vi "AddConstantPotential.vi"(0 "deviceName":string, 1 "channel":u8, 2 "repeats":u16=1, 3 "potential":sgl, 4 "samplingInterval":sgl, 5 "maxDuration":sgl, 6 "isVoltageVsOCP":bool, 7 "error in (no error)":errorcluster, 8 "maxAbsoluteCurrent":sgl=inf, 10 "minAbsoluteCurrent":sgl, 12 "maxCapacity":sgl=inf, 13 "mindIdt":sgl, 14 "approxMaxCurrent":sgl=inf, 15 "isAutoRange":bool=TRUE, 16 "voltageRange":i32=-1) -> (27 "error out":errorcluster)   [LabVIEW 2018]
doc: "EXPORT void AisAddConstantPotential(const char* deviceName, uint8_t channel, uint16_t repeats, float potential, float samplingInterval, float maxDuration, bool isVoltageVsOCP, float maxAbsoluteCurrent, float maxCurrent, float minAbsoluteCurrent, float minCurrent, float maxCapacity, float mindIdt, float approxMaxCurrent, bool isAutoRange, int voltageRange);"
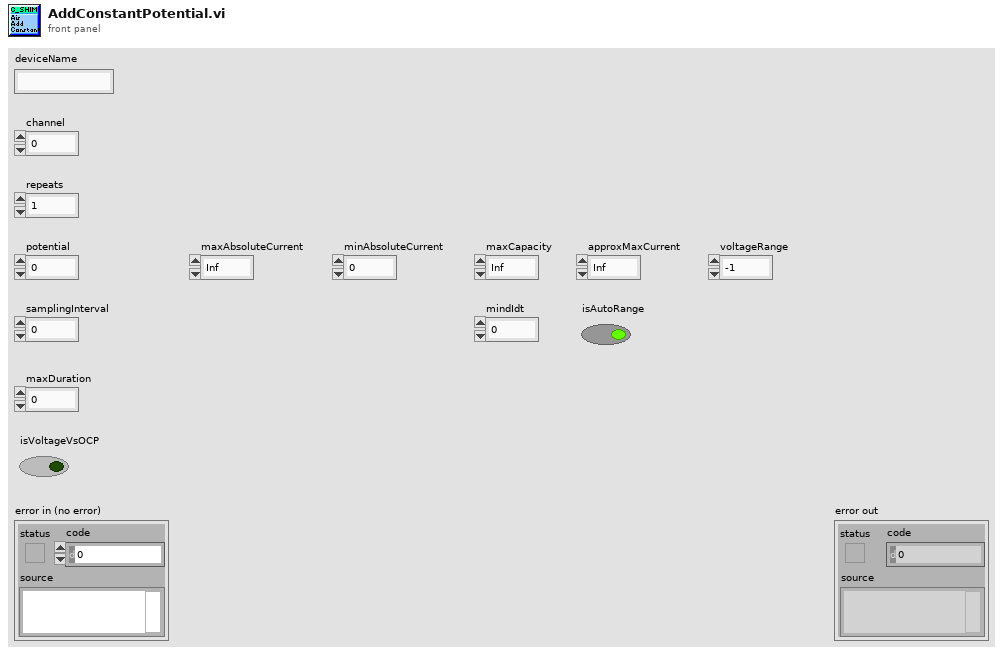
[diagram p1: front panel]
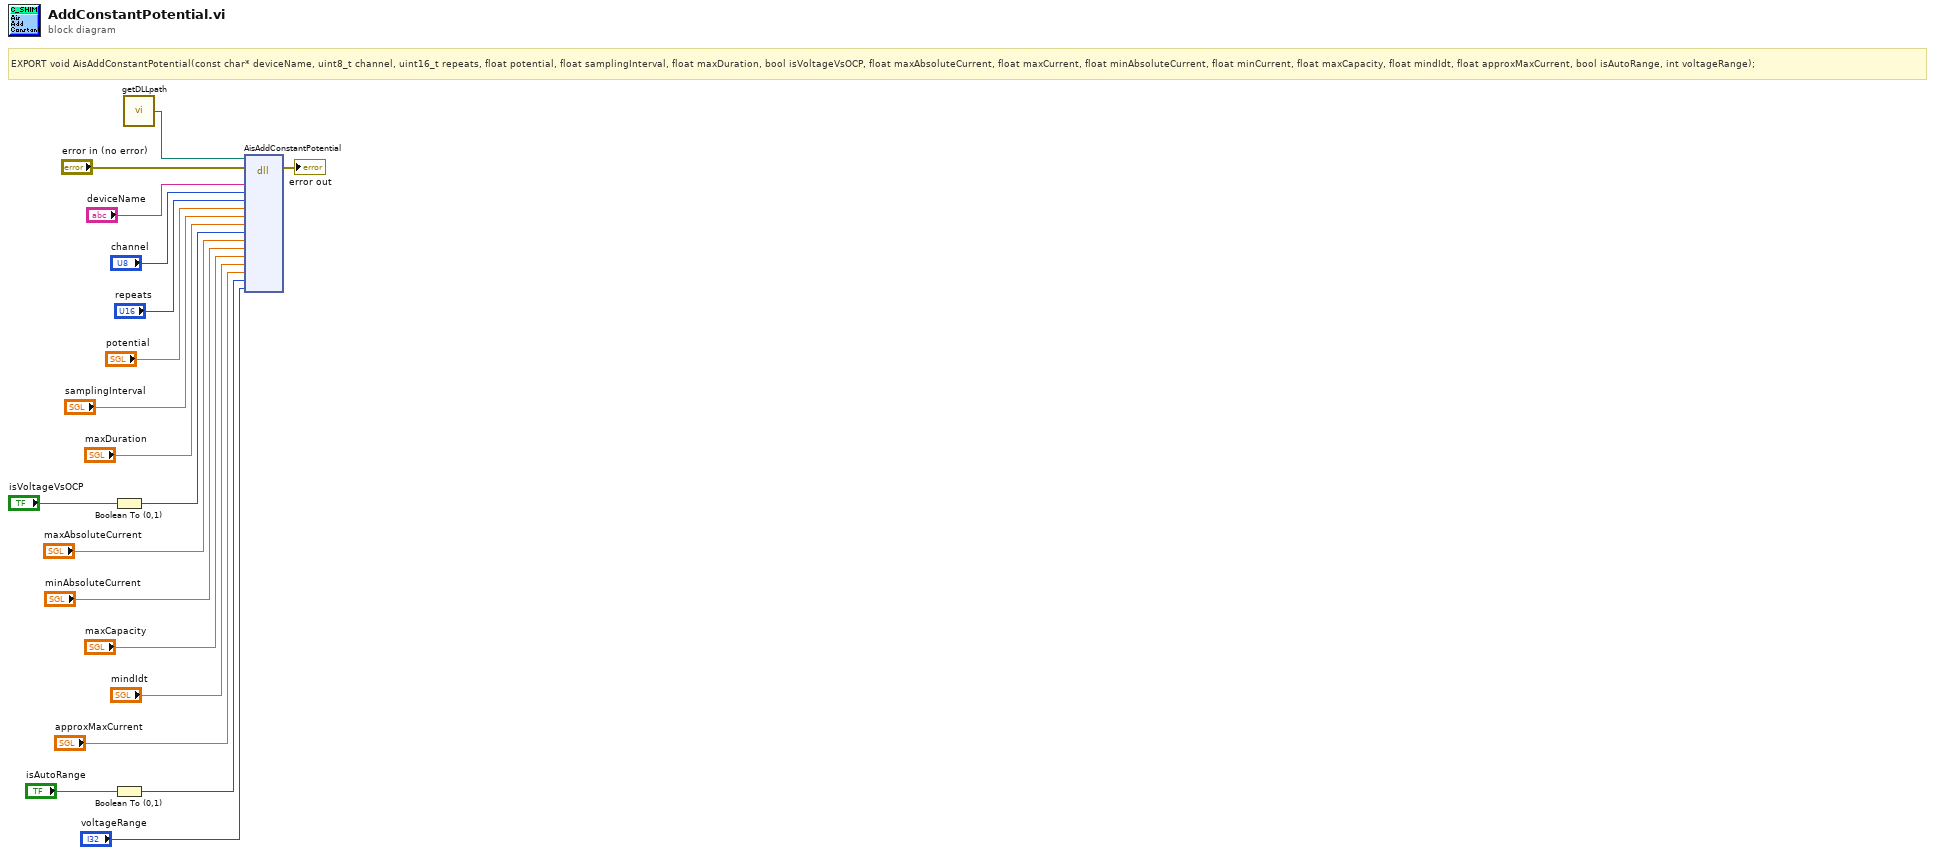
[diagram p0: block diagram]
diagram:
  # "EXPORT void AisAddConstantPotential(const char* deviceName, uint8_t channel, uint16_t repeats, float potential, float samplingInterval, float maxDuration, bool isVoltageVsOCP, float maxAbsoluteCurrent, float maxCurrent, float minAbsoluteCurrent, float minCurrent, float maxCapacity, float mindIdt, float approxMaxCurrent, bool isAutoRange, int voltageRange);"
  n1 = Boolean To (0,1)(Boolean="isVoltageVsOCP") -> (0, 1=w12:i16)
  n2 = Boolean To (0,1)(Boolean="isAutoRange") -> (0, 1=w5:i16)
  n3 = call "getDLLpath.vi"() -> ("DLL_Path"=w1:path)
  n4 = dll-call lib="?" fn="AisAddConstantPotential"(path in=w1, error in="error in (no error)", "deviceName"="deviceName", "channel"="channel", "repeats"="repeats", "potential"="potential", "samplingInterval"="samplingInterval", "maxDuration"="maxDuration", "isVoltageVsOCP"=w12, "maxAbsoluteCurrent"="maxAbsoluteCurrent", "minAbsoluteCurrent"="minAbsoluteCurrent", "maxCapacity"="maxCapacity", "mindIdt"="mindIdt", "approxMaxCurrent"="approxMaxCurrent", "isAutoRange"=w5, "voltageRange"="voltageRange") -> (error out=→"error out":errorcluster)  [unwired: 16 in, 1 out]
